vi "deleteStep.vi"(0 "Script in":T1, 7 "index in":i32) -> (4 "Script out":T1, 6 "index out":i32)   [LabVIEW 2019]
uses:
  TypeDef/Script.ctl
  TypeDef/Step.ctl
  TypeDef/Direction.ctl
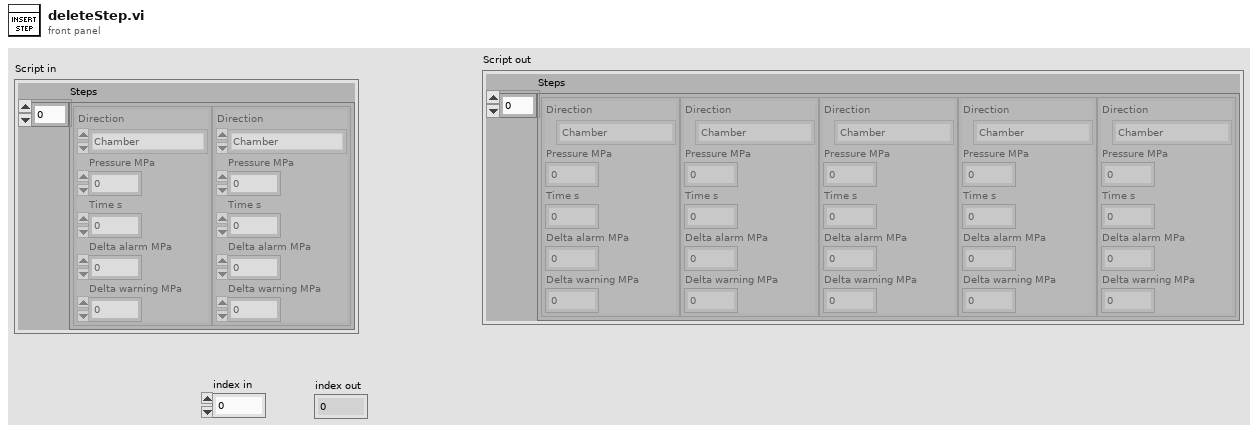
[diagram p1: front panel]
types:
  T1 = typedef "Script.ctl" = cluster{"Steps":T2[]}
  T2 = typedef "Step.ctl" = cluster{"Direction":T3, "Pressure MPa":dbl, "Time s":dbl, "Delta alarm MPa":dbl, "Delta warning MPa":dbl}
  T3 = typedef "Direction.ctl" = enum16{"None", "Chamber", "DUT"}
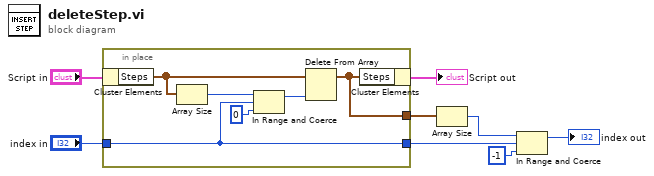
[diagram p0: block diagram]
diagram:
  n1 = in-place {
    in-place-border: [w10] -> w6
    in-place-border: "index in" -> [w9]
    in-place-border: [w9] -> w3
    n2 = in-place-cluster #1("Script in") -> ("Steps"=w13:T2[])
    n3 = Array Size(array=w13) -> (size(s)=w12:i32)
    n4 = In Range and Coerce(upper limit=w12, x=w9, lower limit=0) -> (coerced(x)=w11:i32)  [unwired: 1 out]
    n5 = Delete From Array(array=w13, index=w11) -> (array with subset deleted=w10:T2[])  [unwired: 1 in, 1 out]
    n6 = in-place-cluster #1("Steps"=w10) -> (→"Script out":T1)
  }
  n7 = Array Size(array=w6) -> (size(s)=w4:i32)
  n8 = In Range and Coerce(upper limit=w4, x=w3, lower limit=-1) -> (coerced(x)=→"index out":i32)  [unwired: 1 out]
